vi "name.vi"(8 "error in (no error)":errorcluster, 11 "Coke in":refnum<class "Coke.lvclass">) -> (0 "error out":errorcluster, 2 "name":string, 3 "Coke out":refnum<class "Coke.lvclass">)   [LabVIEW 2017, in "Coke.lvclass"]
uses:
  Coke.lvclass
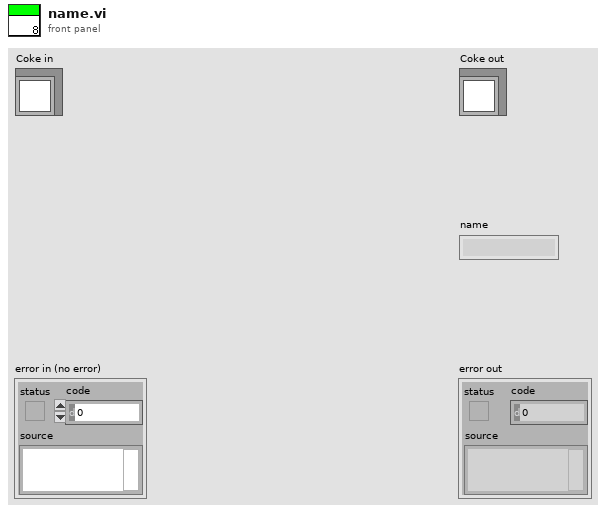
[diagram p1: front panel]
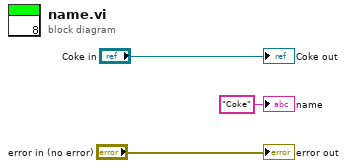
[diagram p0: block diagram]
diagram:
  "error out" <- "error in (no error)"
  "Coke out" <- "Coke in"
  "name" <- "Coke" ("name")
